vi "Spex ScanPar.vi"(0 "Port":refnum<visa-resource-name>="COM1" caption="Com Port", 1 "Scan Type":bool caption="Scan Type  (Burst)", 2 "Count":i32=1 min=1 max=999 step=1, 3 "Delay":dbl caption="Delay (s)" min=0.0 max=600.0 step=0.01 format="%#.3g", 5 "Start(nm)":dbl format="%#.3g", 7 "End(nm)":dbl format="%#.3g", 9 "Rate(nm/s)":dbl=1.0 format="%#.3g", 11 "error in":errorcluster, 12 "Step (nm)":dbl=1.0 min=0.001 max=1000.0 step=0.001 format="%#.3g", 13 "Dwell (s)":dbl min=0.0 max=600.0 step=0.01 format="%#.3g") -> (15 "error out":errorcluster)   [LabVIEW 2010]
uses:
  <vilib>/Instr/_visa.llb/VISA Configure Serial Port (Instr).vi
panel:
  # "Scan parameters"
  # "Continuous"
  # "Burst"
  # "Burst parameters"
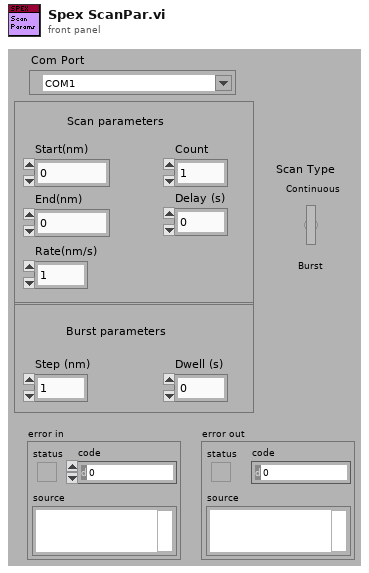
[diagram p1: front panel]
types:
  T1 = enum16{"Send Start", "Send End", "Send Rate", "Send Type", "Send Count", "Send Delay", "Send Step", "Send Dwell", "Wait Answer", "Error/End"}
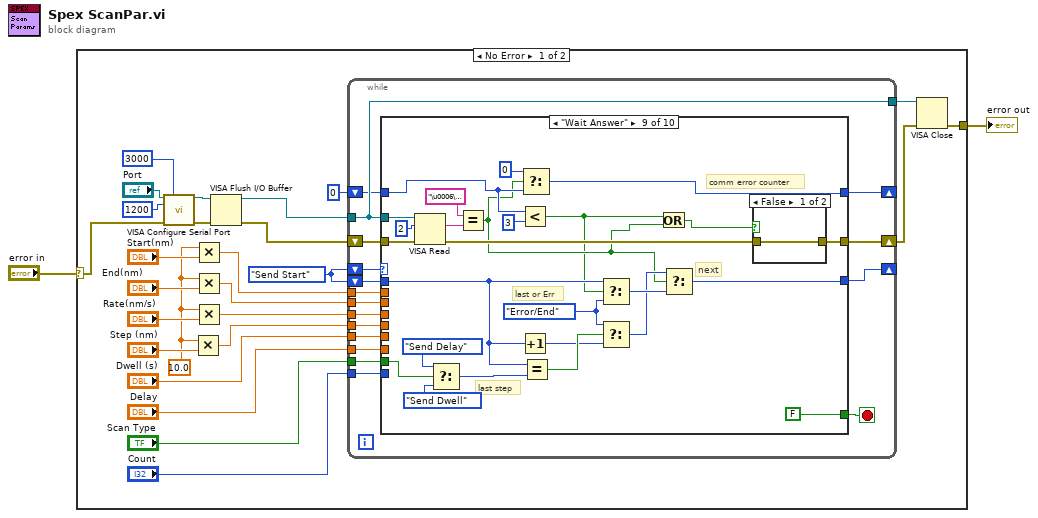
[diagram p0: block diagram]
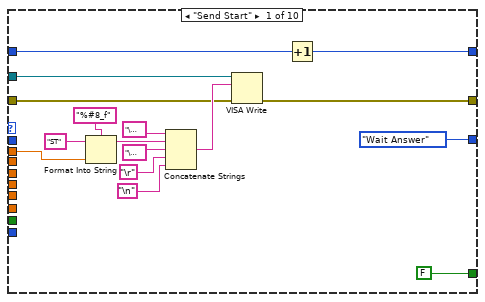
[diagram p2: hidden frame]
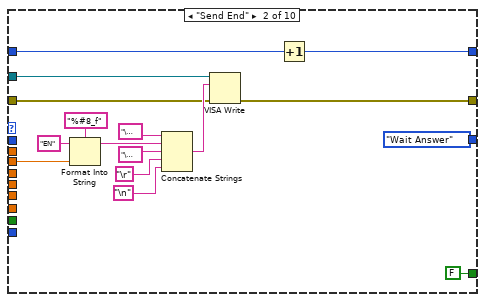
[diagram p3: hidden frame]
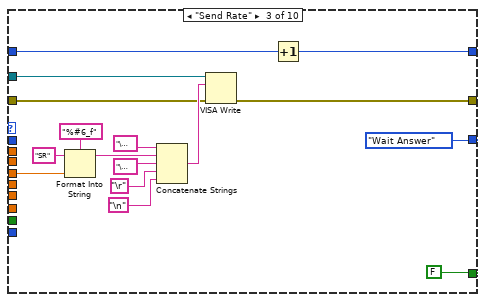
[diagram p4: hidden frame]
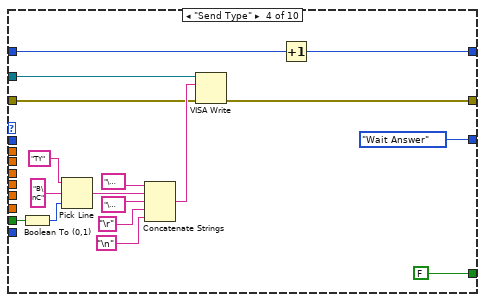
[diagram p5: hidden frame]
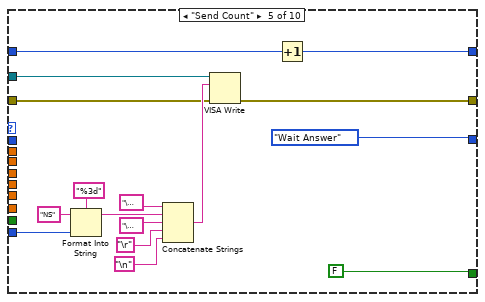
[diagram p6: hidden frame]
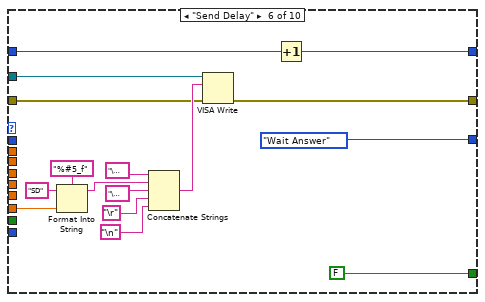
[diagram p7: hidden frame]
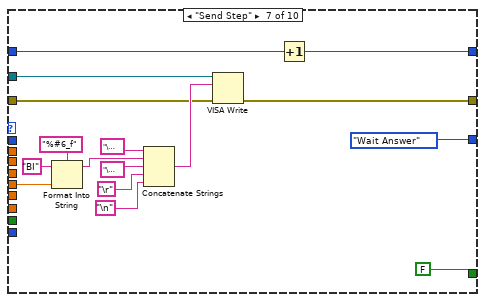
[diagram p8: hidden frame]
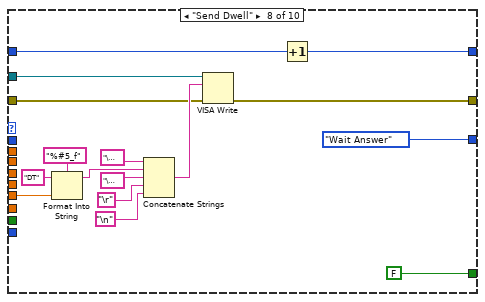
[diagram p9: hidden frame]
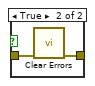
[diagram p10: hidden frame]
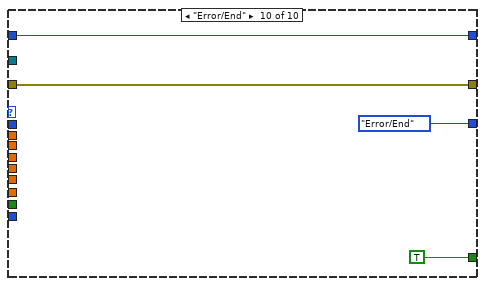
[diagram p11: hidden frame]
diagram:
  n1 = case shown="No Error" "error in" {
    selector: "error in" -> [w3 w208]
    tunnel: [w4 w208] -> w2
    frame No Error {
      w12 = T1."Send Start"
      w7 = 10.0 ("y")
      n2 = call-poly "VISA Configure Serial Port"("VISA resource name"="Port", "timeout (10sec)"=u32 3000, "baud rate (9600)"=u32 1200, "error in (no error)"=w3) -> ("VISA resource name out"=w26:refnum<visa-resource-name>, "error out"=w27:errorcluster)  [unwired: 10 in]
      n3 = Multiply(x=w7, y="Step (nm)") -> (x*y=w13:dbl)
      n4 = Multiply(x=w7, y="Start(nm)") -> (x*y=w21:dbl)
      n5 = Multiply(x=w7, y="End(nm)") -> (x*y=w19:dbl)
      n6 = Multiply(x=w7, y="Rate(nm/s)") -> (x*y=w17:dbl)
      n7 = VISA Flush I/O Buffer(VISA resource name=w26, error in (no error)=w27) -> (VISA resource name out=w24:refnum<visa-resource-name>, error out=w25:errorcluster)  [unwired: 1 in]
      n8 = while {
        shift-right: [w29] -> _
        shift-left: w12 -> [w45]
        tunnel: w24 -> [w40]
        shift-right: [w43] -> w5
        shift-left: w25 -> [w44]
        tunnel: w21 -> [w41]
        tunnel: [w40] -> w23
        shift-right: [w38] -> _
        shift-left: 0 -> [w39]
        shift-left: w12 -> [w37]
        tunnel: w19 -> [w36]
        tunnel: w17 -> [w35]
        tunnel: "Scan Type" -> [w34]
        tunnel: "Count" -> [w33]
        tunnel: "Delay" -> [w32]
        tunnel: w13 -> [w31]
        tunnel: "Dwell (s)" -> [w30]
        stop <- w42 stop-if-true
        n9 = case shown="\"Wait Answer\"" w45 {
          tunnel: w40 -> [w56 w72 w88 w105 w121 w137 w153 w169 w198 _]
          tunnel: w44 -> [w55 w71 w87 w104 w120 w136 w152 w168 w197 w204]
          tunnel: [w54 w70 w86 w103 w119 w135 w151 w167 w179 w204] -> w43
          tunnel: [T1."Wait Answer" T1."Wait Answer" T1."Wait Answer" T1."Wait Answer" T1."Wait Answer" T1."Wait Answer" T1."Wait Answer" T1."Wait Answer" w199 T1."Error/End"] -> w29
          tunnel: [FALSE FALSE FALSE FALSE FALSE FALSE FALSE FALSE FALSE TRUE] -> w42
          tunnel: w41 -> [w50 _ _ _ _ _ _ _ _ _]
          tunnel: w39 -> [w48 w65 w81 w101 w114 w130 w146 w162 w178 w206]
          tunnel: [w47 w64 w80 w100 w113 w129 w145 w161 w191 w206] -> w38
          tunnel: w37 -> [_ _ _ _ _ _ _ _ w187 _]
          tunnel: w36 -> [_ w63 _ _ _ _ _ _ _ _]
          tunnel: w35 -> [_ _ w79 _ _ _ _ _ _ _]
          tunnel: w34 -> [_ _ _ w97 _ _ _ _ w184 _]
          tunnel: w33 -> [_ _ _ _ w112 _ _ _ _ _]
          tunnel: w32 -> [_ _ _ _ _ w128 _ _ _ _]
          tunnel: w31 -> [_ _ _ _ _ _ w144 _ _ _]
          tunnel: w30 -> [_ _ _ _ _ _ _ w160 _ _]
          frame "Send Start" {
            n10 = Format Into String(format string="%#8_f", initial string="ST", w50) -> (resulting string=w49:string)  [unwired: 1 in, 1 out]
            n11 = Concatenate Strings("\u0002" ("string"), w49, "\u0003" ("string"), "\r", "\n") -> (w57:string)
            n12 = VISA Write(VISA resource name=w56, write buffer=w57, error in (no error)=w55) -> (error out=w54:errorcluster)  [unwired: 2 out]
            n13 = Increment(x=w48) -> (x+1=w47:i32)
          }
          frame "Send End" {
            n14 = Format Into String(format string="%#8_f", initial string="EN", w63) -> (resulting string=w66:string)  [unwired: 1 in, 1 out]
            n15 = Concatenate Strings("\u0002" ("string"), w66, "\u0003" ("string"), "\r", "\n") -> (w73:string)
            n16 = VISA Write(VISA resource name=w72, write buffer=w73, error in (no error)=w71) -> (error out=w70:errorcluster)  [unwired: 2 out]
            n17 = Increment(x=w65) -> (x+1=w64:i32)
          }
          frame "Send Rate" {
            n18 = Format Into String(format string="%#6_f", initial string="SR", w79) -> (resulting string=w82:string)  [unwired: 1 in, 1 out]
            n19 = Concatenate Strings("\u0002" ("string"), w82, "\u0003" ("string"), "\r", "\n") -> (w89:string)
            n20 = VISA Write(VISA resource name=w88, write buffer=w89, error in (no error)=w87) -> (error out=w86:errorcluster)  [unwired: 2 out]
            n21 = Increment(x=w81) -> (x+1=w80:i32)
          }
          frame "Send Type" {
            n22 = Boolean To (0,1)(Boolean=w97) -> (0, 1=w96:i16)
            n23 = Pick Line(string ("")="TY" ("initial string"), multi-line string="B\nC", line index=w96) -> (output string=w95:string)
            n24 = Concatenate Strings("\u0002" ("string"), w95, "\u0003" ("string"), "\r", "\n") -> (w106:string)
            n25 = VISA Write(VISA resource name=w105, write buffer=w106, error in (no error)=w104) -> (error out=w103:errorcluster)  [unwired: 2 out]
            n26 = Increment(x=w101) -> (x+1=w100:i32)
          }
          frame "Send Count" {
            n27 = Format Into String(format string="%3d", initial string="NS", w112) -> (resulting string=w115:string)  [unwired: 1 in, 1 out]
            n28 = Concatenate Strings("\u0002" ("string"), w115, "\u0003" ("string"), "\r", "\n") -> (w122:string)
            n29 = VISA Write(VISA resource name=w121, write buffer=w122, error in (no error)=w120) -> (error out=w119:errorcluster)  [unwired: 2 out]
            n30 = Increment(x=w114) -> (x+1=w113:i32)
          }
          frame "Send Delay" {
            n31 = Format Into String(format string="%#5_f", initial string="SD", w128) -> (resulting string=w131:string)  [unwired: 1 in, 1 out]
            n32 = Concatenate Strings("\u0002" ("string"), w131, "\u0003" ("string"), "\r", "\n") -> (w138:string)
            n33 = VISA Write(VISA resource name=w137, write buffer=w138, error in (no error)=w136) -> (error out=w135:errorcluster)  [unwired: 2 out]
            n34 = Increment(x=w130) -> (x+1=w129:i32)
          }
          frame "Send Step" {
            n35 = Format Into String(format string="%#6_f", initial string="BI", w144) -> (resulting string=w147:string)  [unwired: 1 in, 1 out]
            n36 = Concatenate Strings("\u0002" ("string"), w147, "\u0003" ("string"), "\r", "\n") -> (w154:string)
            n37 = VISA Write(VISA resource name=w153, write buffer=w154, error in (no error)=w152) -> (error out=w151:errorcluster)  [unwired: 2 out]
            n38 = Increment(x=w146) -> (x+1=w145:i32)
          }
          frame "Send Dwell" {
            n39 = Format Into String(format string="%#5_f", initial string="DT", w160) -> (resulting string=w163:string)  [unwired: 1 in, 1 out]
            n40 = Concatenate Strings("\u0002" ("string"), w163, "\u0003" ("string"), "\r", "\n") -> (w170:string)
            n41 = VISA Write(VISA resource name=w169, write buffer=w170, error in (no error)=w168) -> (error out=w167:errorcluster)  [unwired: 2 out]
            n42 = Increment(x=w162) -> (x+1=w161:i32)
          }
          frame "Wait Answer" {
            w185 = T1."Error/End"
            # "comm error counter"
            # "last step"
            # "last or Err"
            # "next"
            n43 = VISA Read(VISA resource name=w198, byte count=u32 2, error in (no error)=w197) -> (read buffer=w195:string, error out=w180:errorcluster)  [unwired: 2 out]
            n44 = Select(t=T1."Send Delay", s=w184, f=T1."Send Dwell") -> (s? t:f=w181:T1)
            n45 = Equal?(x="\u0006\u0018", y=w195) -> (x = y?=w177:bool)
            n46 = Less?(x=w178, y=3) -> (x < y?=w176:bool)
            n47 = Increment(x=w187) -> (x+1=w186:T1)
            n48 = Select(t=0, s=w177, f=w178) -> (s? t:f=w191:i32)
            n49 = Equal?(x=w187, y=w181) -> (x = y?=w190:bool)
            n50 = Select(t=w187, s=w176, f=w185) -> (s? t:f=w192:T1)
            n51 = Select(t=w185, s=w190, f=w186) -> (s? t:f=w188:T1)
            n52 = Or(x=w176, y=w177) -> (x .or. y?=w175:bool)
            n53 = Select(t=w188, s=w177, f=w192) -> (s? t:f=w199:T1)
            n54 = case shown="False" w175 {
              tunnel: w180 -> [w201 w203]
              tunnel: [w201 w202] -> w179
              frame False {
              }
              frame True {
                n55 = call <vilib>:"Clear Errors.vi"("error in (no error)"=w203) -> ("error out"=w202:errorcluster)  [unwired: 6 in]
              }
            }
          }
          frame "Error/End" {
          }
        }
      }
      n56 = VISA Close(VISA resource name=w23, error in (no error)=w5) -> (error out=w4:errorcluster)
    }
    frame Error {
    }
  }
  "error out" <- w2
